vi "get module information.vi"(8 "error in":errorcluster, 11 "Module in":refnum<class "Module.lvclass">) -> (0 "error out":errorcluster, 2 "Module Information":T1 {"product ID" format="%.0x"}, 3 "Module out":refnum<class "Module.lvclass">)   [LabVIEW 2014, in "SMI.lvlib" / "Module.lvclass"]
uses:
  Module.lvclass
  module information.ctl
  Device/read serial number.vi
  Device/read product ID.vi
  Device/read product name.vi
  Device/read vendor name.vi
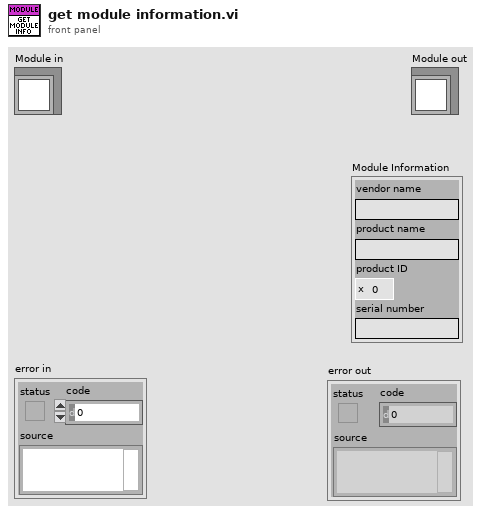
[diagram p1: front panel]
types:
  T1 = typedef "SMI.lvlib/Module.lvclass/module information.ctl" = cluster{"vendor name":string, "product name":string, "product ID":u16, "serial number":string}
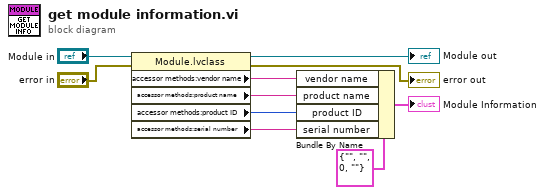
[diagram p0: block diagram]
diagram:
  n1 = property class="Module.lvclass"(reference="Module in", error in="error in") -> (reference out=→"Module out":refnum<class "Module.lvclass">, error out=→"error out":errorcluster, "accessor methods:vendor name"=w6:string, "accessor methods:product name"=w5:string, "accessor methods:product ID"=w1:u16, "accessor methods:serial number"=w4:string)
  n2 = Bundle By Name(cluster=T1 {"vendor name"="", "product name"="", "product ID"=0, "serial number"=""} ("Module Information"), "vendor name"=w6, "product name"=w5, "product ID"=w1, "serial number"=w4) -> (→"Module Information":T1)
